vi "state machine.vi"() -> ()   [LabVIEW 2017]
uses:
  <vilib>/rvi/Emulation/niFpgaGetClockAttributes.vi
  <vilib>/rvi/Emulation/niFpgaSctlEmulationGetInTimedLoop.vi
  <vilib>/rvi/Emulation/niFpgaEmulationReportErrorSimple.vi
  <vilib>/rvi/Emulation/niFpgaProcessEmulError.vi
  <vilib>/rvi/interface/RandomDataEmulation/niFpgaRandomDataHandleErrors.vi
  <vilib>/rvi/eio/common/nirviEmuTemplateMethod_errors.vi
  <vilib>/rvi/Emulation/niFpgaCriticalErrorInLSC.vi
  <vilib>/rvi/DataTransferAndStorage/Container/XNode/niFpgaContainer.xnode
  <vilib>/rvi/interface/RandomDataEmulation/nirviRandomDataFpgaReadWriteTemplate.vi
  <vilib>/eio/EIONode/EIONode.xnode
panel:
  out "real-time port D monitor":bool[](array[boolean])
  out "real-time port C monitor":bool[](array[boolean])
  out "real-time port B monitor":bool[](array[boolean])
  out "real-time port A monitor":bool[](array[boolean])
  in  "stop":bool
  out "reset LED":bool
  out "run LED":bool
  in  "Reset":bool
  out "load LED":bool
  out "idle LED":bool
  in  "Run":bool
  in  "Load":bool
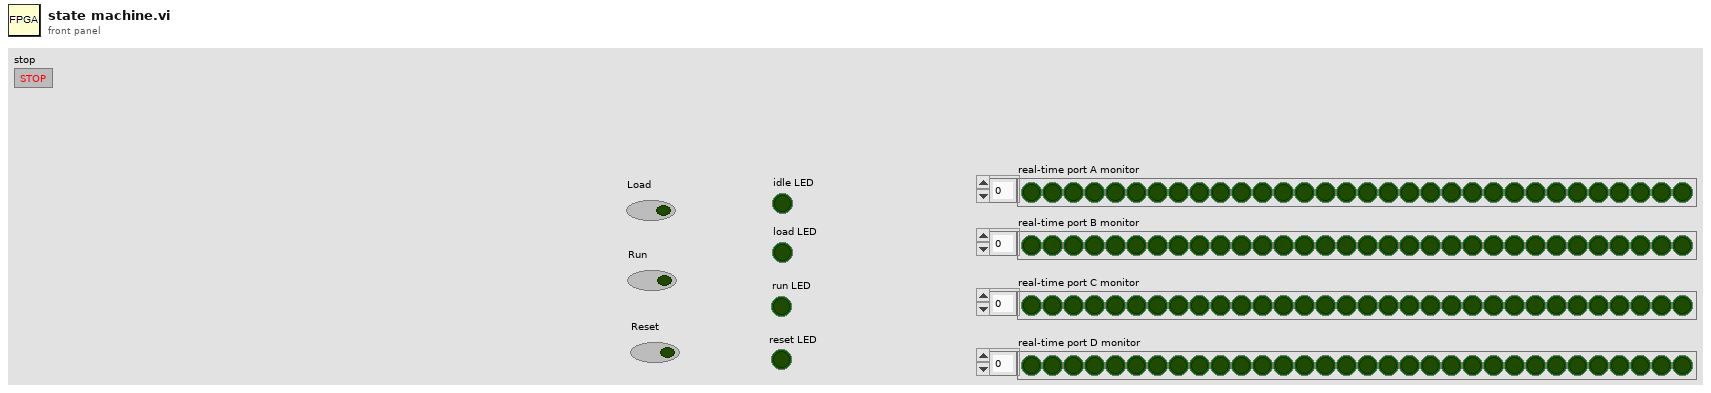
[diagram p1: front panel]
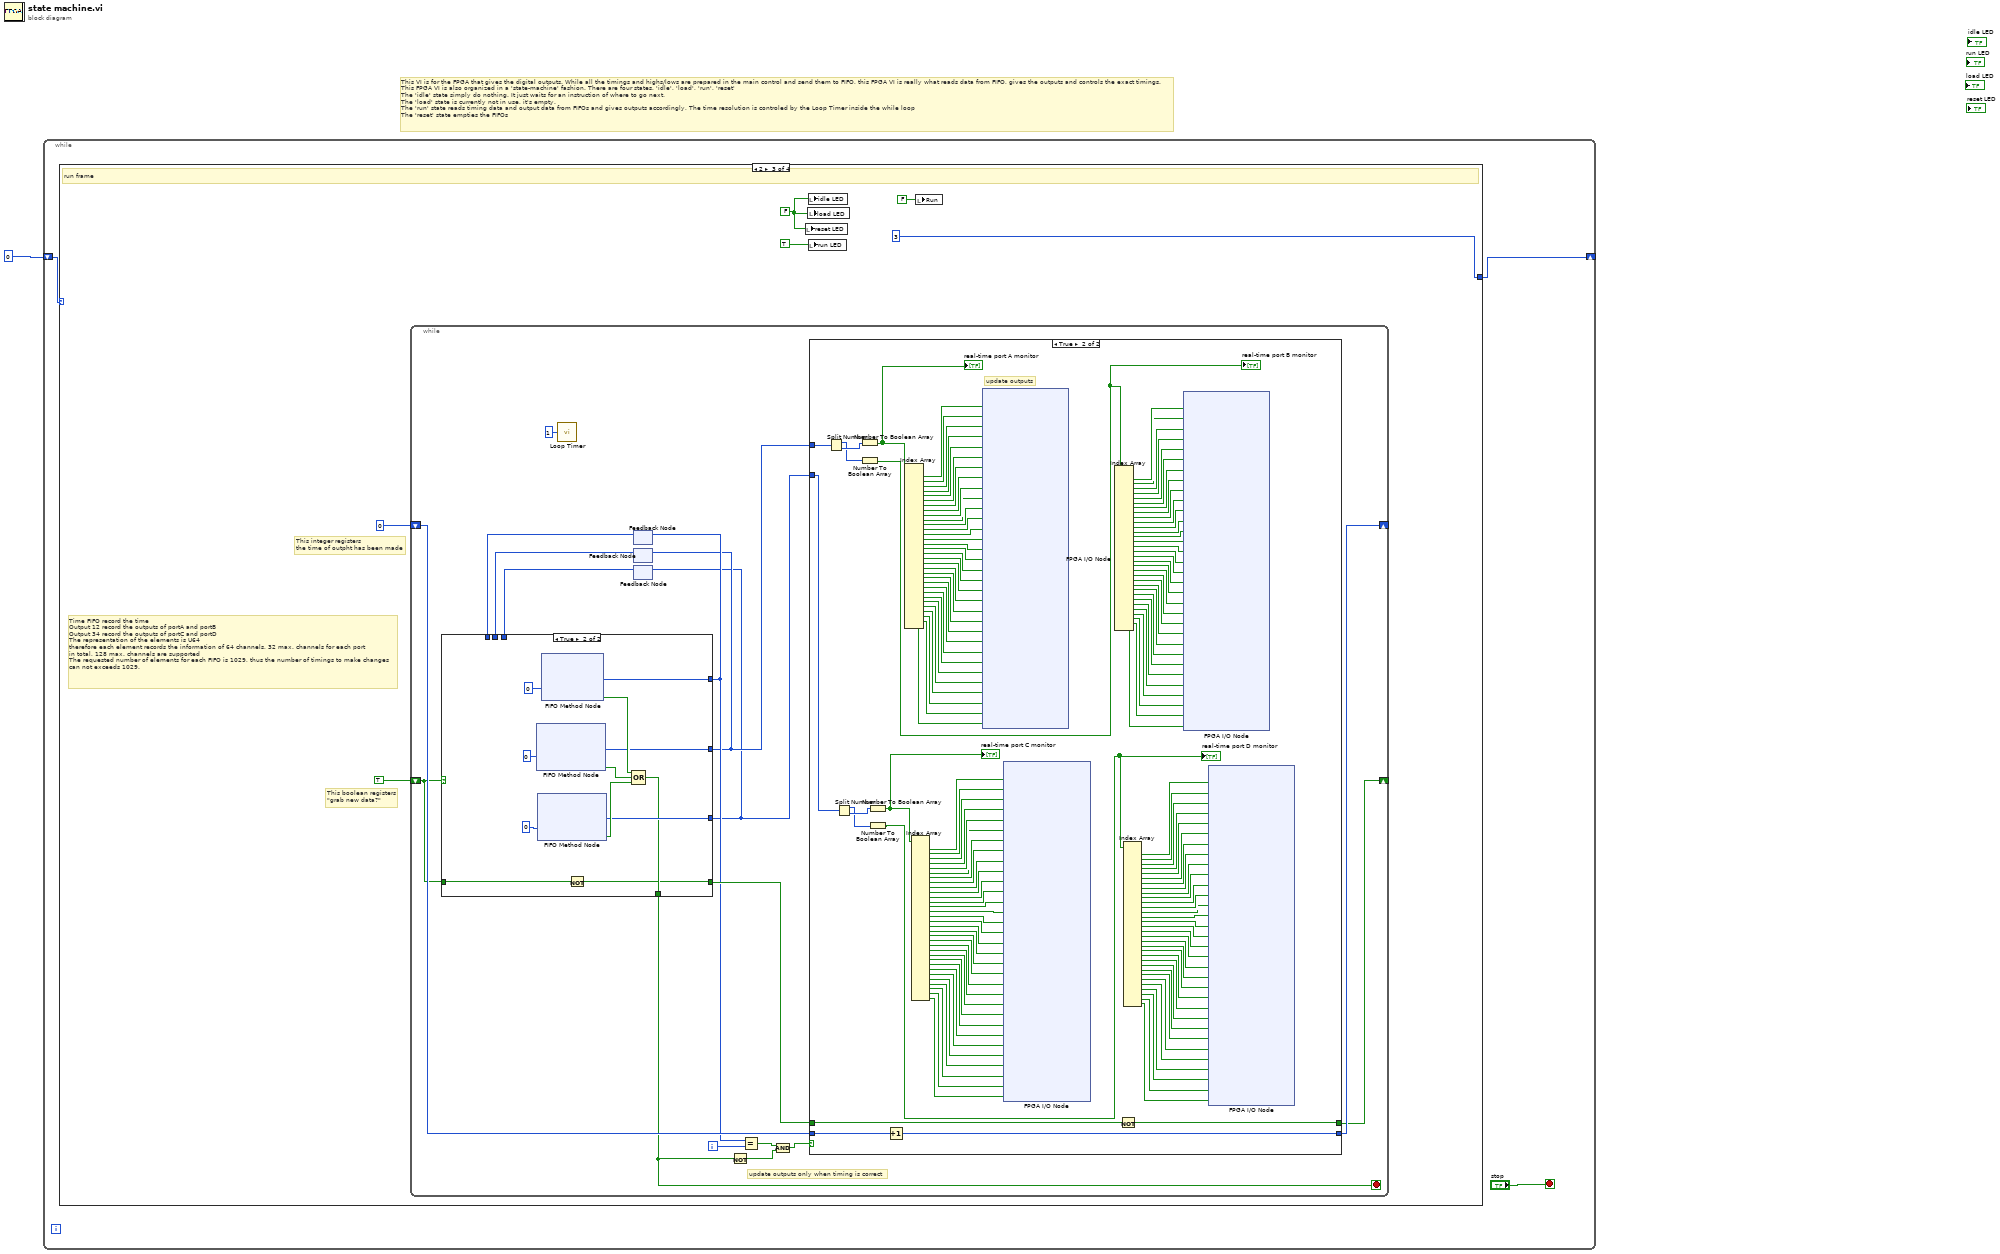
[diagram p0: block diagram]
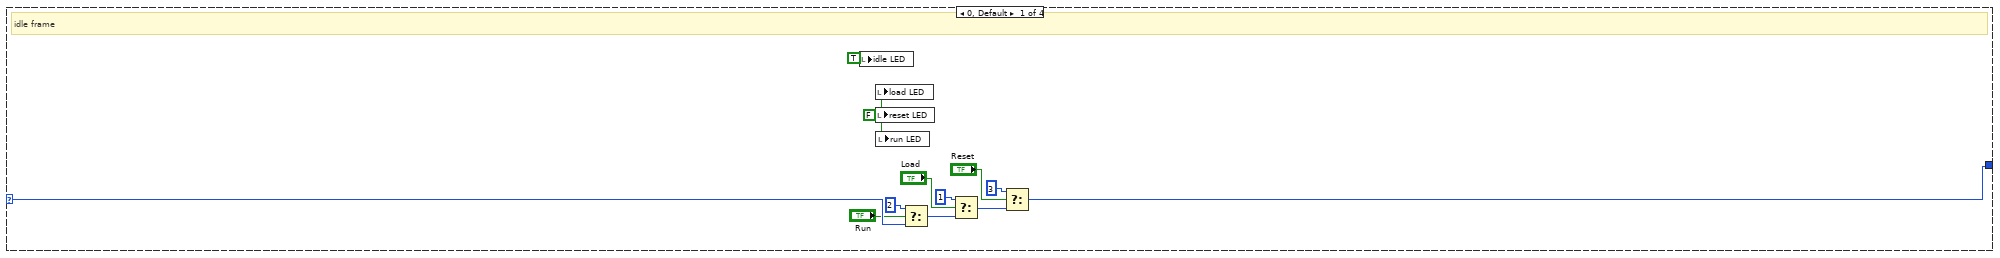
[diagram p2: hidden frame]
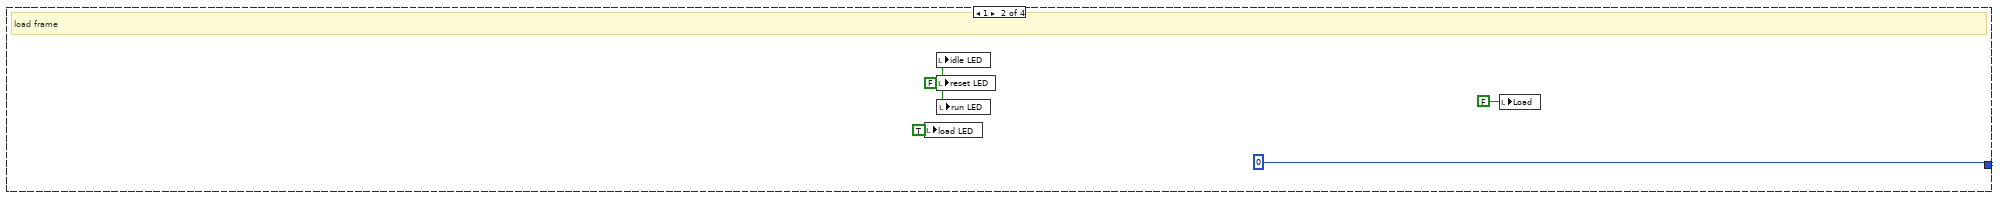
[diagram p3: hidden frame]
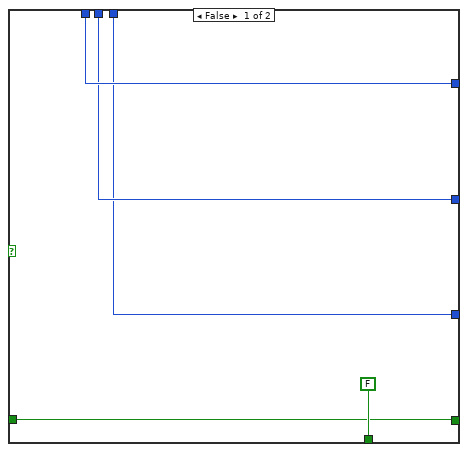
[diagram p4: hidden frame]
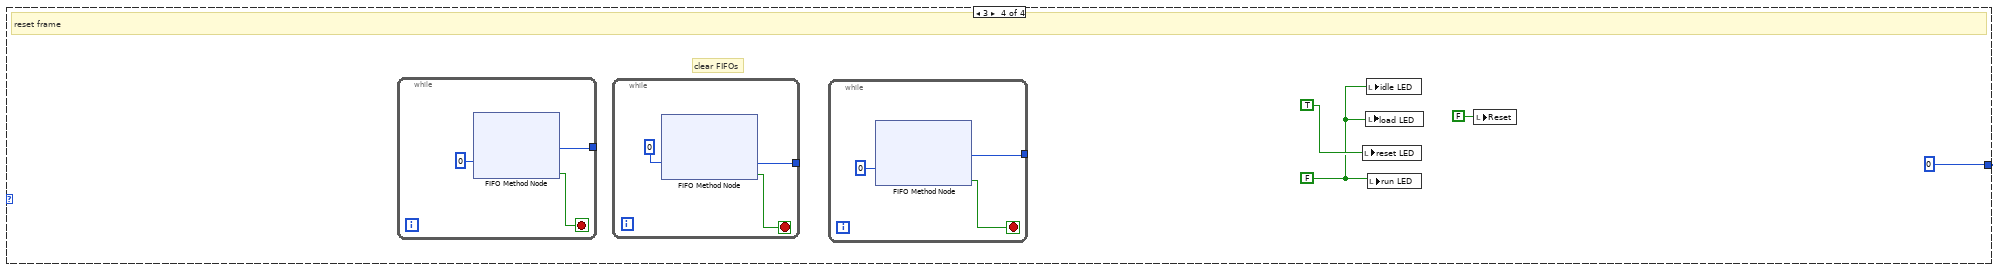
[diagram p6: hidden frame]
diagram:
  # "This VI is for the FPGA that gives the digital outputs. While all the timings and highs/lows are prepared in the main control and send them to FIFO, this FPGA VI is really what reads data from FIFO, gives the outputs and controls the exact timings.\nThis FPGA VI is also organized in a 'state-machine' fashion. There are four states, 'idle', 'load', 'run', 'reset'\nThe 'idle' state simply do nothing. It just waits for an instruction of where to go next.\nThe 'load' state is currently not in use, it's empty.\nThe 'run' state reads timing data and output data from FIFOs and gives outputs accordingly, The time resolution is controled by the Loop Timer inside the while loop\nThe 'reset' state empties the FIFOs"
  n1 = while {
    shift-right: [w3] -> _
    shift-left: i16 0 -> [w4]
    stop <- "stop" stop-if-true
    n2 = case shown="2" w4 {
      selector: w4 -> [w14 _ _ _]
      tunnel: [w7 i16 0 i16 3 i16 0] -> w3
      frame 0, Default {
        w15 = FALSE ("run")
        # "idle frame"
        n3 = local write "idle LED"(TRUE ("run")) -> ()
        n4 = local write "load LED"(w15) -> ()
        n5 = local write "reset LED"(w15) -> ()
        n6 = local write "run LED"(w15) -> ()
        n7 = Select(t=i16 2, s="Run", f=w14) -> (s? t:f=w11:i16)
        n8 = Select(t=i16 1, s="Load", f=w11) -> (s? t:f=w9:i16)
        n9 = Select(t=i16 3, s="Reset", f=w9) -> (s? t:f=w7:i16)
      }
      frame 1 {
        w20 = FALSE ("run")
        # "load frame"
        n10 = local write "load LED"(TRUE ("load")) -> ()
        n11 = local write "idle LED"(w20) -> ()
        n12 = local write "reset LED"(w20) -> ()
        n13 = local write "run LED"(w20) -> ()
        n14 = local write "Load"(FALSE) -> ()
      }
      frame 2 {
        w25 = FALSE ("run")
        # "This integer registers \nthe time of outpht has been made"
        # "This boolean registers\n\"grab new data?\""
        # "Time FIFO record the time\nOutput 12 record the outputs of portA and portB\nOutput 34 record the outputs of portC and portD\nThe representation of the elements is U64\ntherefore each element records the information of 64 channels, 32 max. channels for each port\nin total, 128 max. channels are supported\nThe requested number of elements for each FIFO is 1029, thus the number of timings to make changes \ncan not exceeds 1029."
        # "run frame"
        n15 = while {
          shift-right: [w41] -> _
          shift-left: i16 0 -> [w42]
          shift-right: [w35] -> _
          shift-left: TRUE ("Boolean") -> [w34]
          i -> [w43]
          stop <- w38 stop-if-true
          # "update outputs only when timing is correct"
          n16 = call "Loop Timer"("Count(uSec)"=u8 1) -> ()  [unwired: 1 out]
          n17 = feedback #1() -> (w30:u64)  [unwired: 1 in]
          n18 = feedback #2() -> (w29:u64)  [unwired: 1 in]
          n19 = feedback #3() -> (w28:u64)  [unwired: 1 in]
          n20 = case shown="True" w34 {
            tunnel: [w45 w54] -> w32
            tunnel: [w44 w53] -> w31
            tunnel: [w46 w52] -> w33
            tunnel: [FALSE w51] -> w38
            tunnel: w34 -> [w47 w50]
            tunnel: [w47 w49] -> w36
            tunnel: w30 -> [w46 _]
            tunnel: w29 -> [w45 _]
            tunnel: w28 -> [w44 _]
            frame False {
            }
            frame True {
              n21 = xnode ("FIFO Method Node")("Timeout"=0) -> ("Element"=w54:u64, "Timed Out?"=w55:bool)  [unwired: 1 in, 1 out]
              n22 = xnode ("FIFO Method Node")("Timeout"=0) -> ("Element"=w53:u64, "Timed Out?"=w56:bool)  [unwired: 1 in, 1 out]
              n23 = xnode ("FIFO Method Node")("Timeout"=0) -> ("Element"=w52:u64, "Timed Out?"=w60:bool)  [unwired: 1 in, 1 out]
              n24 = Not(x=w50) -> (.not. x?=w49:bool)
              n25 = Compound Arithmetic op=OR(w60, w55, w56) -> (w51:bool)
            }
          }
          n26 = feedback-in #1(w33) -> ()
          n27 = feedback-in #2(w32) -> ()
          n28 = feedback-in #3(w31) -> ()
          n29 = Not(x=w38) -> (.not. x?=w37:bool)
          n30 = Equal?(x=w33, y=w43) -> (x = y?=w39:bool)
          n31 = And(x=w39, y=w37) -> (x .and. y?=w40:bool)
          n32 = case shown="True" w40 {
            tunnel: w32 -> [_ w152]
            tunnel: w31 -> [_ w91]
            tunnel: w42 -> [w62 w204]
            tunnel: [w62 w203] -> w41
            tunnel: w36 -> [w61 w97]
            tunnel: [w61 w96] -> w35
            frame False {
            }
            frame True {
              # "update outputs"
              n33 = Split Number(x=w152) -> (hi(x)=w94:u32, lo(x)=w95:u32)
              n34 = Split Number(x=w91) -> (hi(x)=w92:u32, lo(x)=w93:u32)
              n35 = Number To Boolean Array(number=w95) -> (Boolean array=w90:bool[])
              "real-time port A monitor" <- w90
              n36 = Number To Boolean Array(number=w94) -> (Boolean array=w87:bool[])
              "real-time port B monitor" <- w87
              n37 = Number To Boolean Array(number=w93) -> (Boolean array=w89:bool[])
              "real-time port C monitor" <- w89
              n38 = Number To Boolean Array(number=w92) -> (Boolean array=w88:bool[])
              "real-time port D monitor" <- w88
              n39 = Increment(x=w204) -> (x+1=w203:i16)
              n40 = Index Array(array=w90) -> (element #1=w202:bool, element #2=w201:bool, element #3=w200:bool, element #4=w199:bool, element #5=w198:bool, element #6=w197:bool, element #7=w196:bool, element #8=w195:bool, element #9=w194:bool, element #10=w193:bool, element #11=w192:bool, element #12=w191:bool, element #13=w190:bool, element #14=w189:bool, element #15=w188:bool, element #16=w187:bool, element #17=w186:bool, element #18=w185:bool, element #19=w184:bool, element #20=w183:bool, element #21=w182:bool, element #22=w181:bool, element #23=w180:bool, element #24=w179:bool, element #25=w178:bool, element #26=w125:bool, element #27=w86:bool, element #28=w85:bool, element #29=w84:bool, element #30=w83:bool, element #31=w82:bool, element #32=w81:bool)  [unwired: 32 in]
              n41 = Index Array(array=w89) -> (element #1=w151:bool, element #2=w149:bool, element #3=w148:bool, element #4=w147:bool, element #5=w146:bool, element #6=w145:bool, element #7=w144:bool, element #8=w143:bool, element #9=w142:bool, element #10=w141:bool, element #11=w140:bool, element #12=w139:bool, element #13=w138:bool, element #14=w137:bool, element #15=w136:bool, element #16=w135:bool, element #17=w134:bool, element #18=w133:bool, element #19=w132:bool, element #20=w131:bool, element #21=w130:bool, element #22=w129:bool, element #23=w128:bool, element #24=w127:bool, element #25=w126:bool, element #26=w123:bool, element #27=w68:bool, element #28=w67:bool, element #29=w66:bool, element #30=w65:bool, element #31=w64:bool, element #32=w63:bool)  [unwired: 32 in]
              n42 = xnode "FPGA I/O Node"("Connector0/DIO0"=w202, "Connector0/DIO1"=w201, "Connector0/DIO2"=w200, "Connector0/DIO3"=w199, "Connector0/DIO4"=w198, "Connector0/DIO5"=w197, "Connector0/DIO6"=w196, "Connector0/DIO7"=w195, "Connector0/DIO8"=w194, "Connector0/DIO9"=w193, "Connector0/DIO10"=w192, "Connector0/DIO11"=w191, "Connector0/DIO12"=w190, "Connector0/DIO13"=w189, "Connector0/DIO14"=w188, "Connector0/DIO15"=w187, "Connector0/DIO16"=w186, "Connector0/DIO17"=w185, "Connector0/DIO18"=w184, "Connector0/DIO19"=w183, "Connector0/DIO20"=w182, "Connector0/DIO21"=w181, "Connector0/DIO22"=w180, "Connector0/DIO23"=w179, "Connector0/DIO24"=w178, "Connector0/DIO25"=w125, "Connector0/DIO26"=w86, "Connector0/DIO27"=w85, "Connector0/DIO28"=w84, "Connector0/DIO29"=w83, "Connector0/DIO30"=w82, "Connector0/DIO31"=w81) -> ()  [unwired: 32 in, 32 out]
              n43 = xnode "FPGA I/O Node"("Connector2/DIO0"=w151, "Connector2/DIO1"=w149, "Connector2/DIO2"=w148, "Connector2/DIO3"=w147, "Connector2/DIO4"=w146, "Connector2/DIO5"=w145, "Connector2/DIO6"=w144, "Connector2/DIO7"=w143, "Connector2/DIO8"=w142, "Connector2/DIO9"=w141, "Connector2/DIO10"=w140, "Connector2/DIO11"=w139, "Connector2/DIO12"=w138, "Connector2/DIO13"=w137, "Connector2/DIO14"=w136, "Connector2/DIO15"=w135, "Connector2/DIO16"=w134, "Connector2/DIO17"=w133, "Connector2/DIO18"=w132, "Connector2/DIO19"=w131, "Connector2/DIO20"=w130, "Connector2/DIO21"=w129, "Connector2/DIO22"=w128, "Connector2/DIO23"=w127, "Connector2/DIO24"=w126, "Connector2/DIO25"=w123, "Connector2/DIO26"=w68, "Connector2/DIO27"=w67, "Connector2/DIO28"=w66, "Connector2/DIO29"=w65, "Connector2/DIO30"=w64, "Connector2/DIO31"=w63) -> ()  [unwired: 32 in, 32 out]
              n44 = Index Array(array=w87) -> (element #1=w177:bool, element #2=w176:bool, element #3=w175:bool, element #4=w174:bool, element #5=w173:bool, element #6=w172:bool, element #7=w171:bool, element #8=w170:bool, element #9=w169:bool, element #10=w168:bool, element #11=w167:bool, element #12=w166:bool, element #13=w165:bool, element #14=w164:bool, element #15=w163:bool, element #16=w162:bool, element #17=w161:bool, element #18=w160:bool, element #19=w159:bool, element #20=w158:bool, element #21=w157:bool, element #22=w156:bool, element #23=w155:bool, element #24=w154:bool, element #25=w153:bool, element #26=w124:bool, element #27=w80:bool, element #28=w79:bool, element #29=w78:bool, element #30=w77:bool, element #31=w76:bool, element #32=w75:bool)  [unwired: 32 in]
              n45 = Not(x=w97) -> (.not. x?=w96:bool)
              n46 = Index Array(array=w88) -> (element #1=w150:bool, element #2=w122:bool, element #3=w121:bool, element #4=w120:bool, element #5=w119:bool, element #6=w118:bool, element #7=w117:bool, element #8=w116:bool, element #9=w115:bool, element #10=w114:bool, element #11=w113:bool, element #12=w112:bool, element #13=w111:bool, element #14=w110:bool, element #15=w109:bool, element #16=w108:bool, element #17=w107:bool, element #18=w106:bool, element #19=w105:bool, element #20=w104:bool, element #21=w103:bool, element #22=w102:bool, element #23=w101:bool, element #24=w100:bool, element #25=w99:bool, element #26=w98:bool, element #27=w74:bool, element #28=w73:bool, element #29=w72:bool, element #30=w71:bool, element #31=w70:bool, element #32=w69:bool)  [unwired: 32 in]
              n47 = xnode "FPGA I/O Node"("Connector1/DIO0"=w177, "Connector1/DIO1"=w176, "Connector1/DIO2"=w175, "Connector1/DIO3"=w174, "Connector1/DIO4"=w173, "Connector1/DIO5"=w172, "Connector1/DIO6"=w171, "Connector1/DIO7"=w170, "Connector1/DIO8"=w169, "Connector1/DIO9"=w168, "Connector1/DIO10"=w167, "Connector1/DIO11"=w166, "Connector1/DIO12"=w165, "Connector1/DIO13"=w164, "Connector1/DIO14"=w163, "Connector1/DIO15"=w162, "Connector1/DIO16"=w161, "Connector1/DIO17"=w160, "Connector1/DIO18"=w159, "Connector1/DIO19"=w158, "Connector1/DIO20"=w157, "Connector1/DIO21"=w156, "Connector1/DIO22"=w155, "Connector1/DIO23"=w154, "Connector1/DIO24"=w153, "Connector1/DIO25"=w124, "Connector1/DIO26"=w80, "Connector1/DIO27"=w79, "Connector1/DIO28"=w78, "Connector1/DIO29"=w77, "Connector1/DIO30"=w76, "Connector1/DIO31"=w75) -> ()  [unwired: 32 in, 32 out]
              n48 = xnode "FPGA I/O Node"("Connector3/DIO0"=w150, "Connector3/DIO1"=w122, "Connector3/DIO2"=w121, "Connector3/DIO3"=w120, "Connector3/DIO4"=w119, "Connector3/DIO5"=w118, "Connector3/DIO6"=w117, "Connector3/DIO7"=w116, "Connector3/DIO8"=w115, "Connector3/DIO9"=w114, "Connector3/DIO10"=w113, "Connector3/DIO11"=w112, "Connector3/DIO12"=w111, "Connector3/DIO13"=w110, "Connector3/DIO14"=w109, "Connector3/DIO15"=w108, "Connector3/DIO16"=w107, "Connector3/DIO17"=w106, "Connector3/DIO18"=w105, "Connector3/DIO19"=w104, "Connector3/DIO20"=w103, "Connector3/DIO21"=w102, "Connector3/DIO22"=w101, "Connector3/DIO23"=w100, "Connector3/DIO24"=w99, "Connector3/DIO25"=w98, "Connector3/DIO26"=w74, "Connector3/DIO27"=w73, "Connector3/DIO28"=w72, "Connector3/DIO29"=w71, "Connector3/DIO30"=w70, "Connector3/DIO31"=w69) -> ()  [unwired: 32 in, 32 out]
            }
          }
        }
        n49 = local write "reset LED"(w25) -> ()
        n50 = local write "load LED"(w25) -> ()
        n51 = local write "idle LED"(w25) -> ()
        n52 = local write "run LED"(TRUE ("run")) -> ()
        n53 = local write "Run"(FALSE) -> ()
      }
      frame 3 {
        w207 = FALSE ("run")
        # "clear FIFOs"
        # "reset frame"
        n54 = while {
          tunnel: [w217] -> _
          stop <- w215 stop-if-true
          n55 = xnode ("FIFO Method Node")("Timeout"=0) -> ("Element"=w217:u64, "Timed Out?"=w215:bool)  [unwired: 1 in, 1 out]
        }
        n56 = while {
          tunnel: [w212] -> _
          stop <- w213 stop-if-true
          n57 = xnode ("FIFO Method Node")("Timeout"=0) -> ("Element"=w212:u64, "Timed Out?"=w213:bool)  [unwired: 1 in, 1 out]
        }
        n58 = while {
          tunnel: [w209] -> _
          stop <- w210 stop-if-true
          n59 = xnode ("FIFO Method Node")("Timeout"=0) -> ("Element"=w209:u64, "Timed Out?"=w210:bool)  [unwired: 1 in, 1 out]
        }
        n60 = local write "reset LED"(TRUE ("run")) -> ()
        n61 = local write "load LED"(w207) -> ()
        n62 = local write "idle LED"(w207) -> ()
        n63 = local write "run LED"(w207) -> ()
        n64 = local write "Reset"(FALSE) -> ()
      }
    }
  }
